vi "SetPosition.vi"(4 "Mode":i32(ring) items=["MoveToPosition", "MoveToLimitAndDefinePosition", "DefinePosition"], 5 "Axis":string="Horizontal Rotator", 6 "Speed":dbl=5.0, 7 "Position":dbl, 8 "error in (no error)":errorcluster, 9 "Instrument Ref In":refnum<k24>) -> (0 "SetPosition Error":i32, 2 "error out":errorcluster, 3 "Instrument Ref Out":refnum<k24>)   [LabVIEW 2019]
uses:
  QDInstrument_LabView (1)/QDInstrument.dll
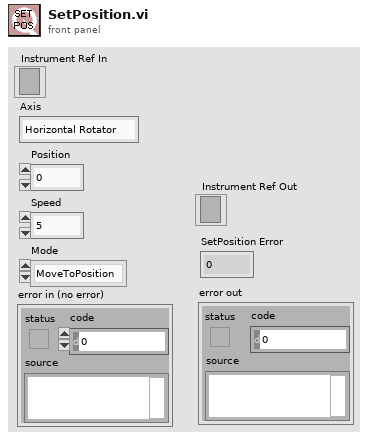
[diagram p1: front panel]
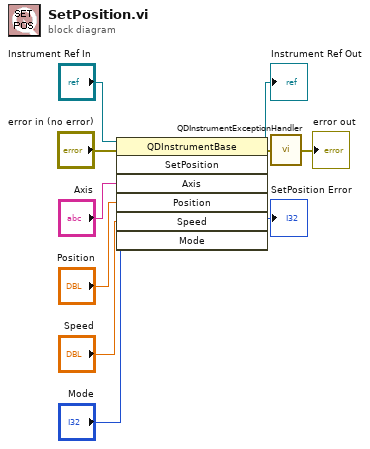
[diagram p0: block diagram]
diagram:
  n1 = invoke class="QDInstrumentBase" method="SetPosition"(reference="Instrument Ref In", error in="error in (no error)", "Axis"="Axis", "Position"="Position", "Speed"="Speed", "Mode"="Mode") -> (reference out=→"Instrument Ref Out":refnum<k24>, error out=w6:errorcluster, "SetPosition"=→"SetPosition Error":i32)  [unwired: 1 in, 4 out]
  n2 = call "QDInstrumentExceptionHandler.vi"("Error in"=w6) -> ("Error out"=→"error out":errorcluster)
